vi "Open TextDocument.vi"(7 "ooWriter":refnum<class "ooWriter.lvclass">, 8 "error in (no error)":errorcluster, 11 "filepath":path) -> (0 "error out":errorcluster, 3 "ooWriter out":refnum<class "ooWriter.lvclass">)   [LabVIEW 2009, in "ooWriter.lvclass"]
uses:
  ooWriter.lvclass
  C:/Projets/LAVAG/OpenOfficeRGT/AODL/DLLs/AODL.dll
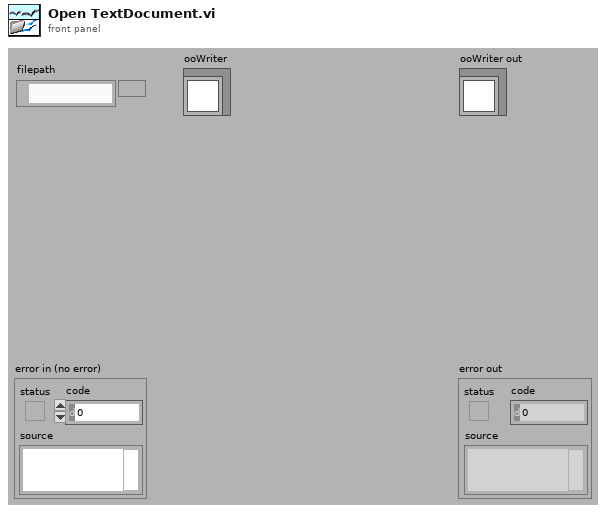
[diagram p1: front panel]
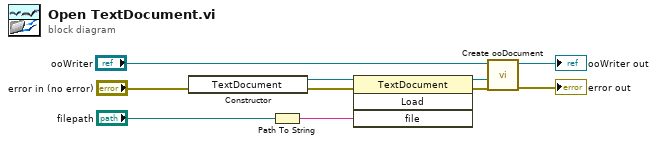
[diagram p0: block diagram]
diagram:
  n1 = constructor class="TextDocument"(error in="error in (no error)") -> (reference out=w10:refnum<k24>, error out=w8:errorcluster)  [unwired: 2 in, 1 out]
  n2 = Path To String(path="filepath") -> (string=w2:string)
  n3 = invoke class="TextDocument" method="Load"(reference=w10, error in=w8, "file"=w2) -> (reference out=w9:refnum<k24>, error out=w7:errorcluster)  [unwired: 1 in, 2 out]
  n4 = call-dynamic "Create ooDocument.vi"("error in (no error)"=w7, "Document"=w9, "ooDocument in"="ooWriter") -> ("error out"=→"error out":errorcluster, "ooDocument out"=→"ooWriter out":refnum<class "ooWriter.lvclass">)  [unwired: 7 in]
